vi "Slack OAuth Test.vi"() -> ()   [LabVIEW 2020]
uses:
  Oauth2.Slack/Oauth2.Slack.lvclass
  C:/Data/1_Projects/CIGH_Oauth2/source/Oauth2/Oauth2.lvclass
  Oauth2/Oauth2.lvclass
  <vilib>/LabVIEW Open Source Project/OpenURI/uri/URI.lvclass
  <vilib>/httpClient/LabVIEWHTTPClient.lvlib
panel:
  out "Slack User List":string
  out "HTTP Response Headers":string
  in  "Client Secret":string
  in  "Client ID":string
  out "Slack Access Token":string
  out "error out":errorcluster
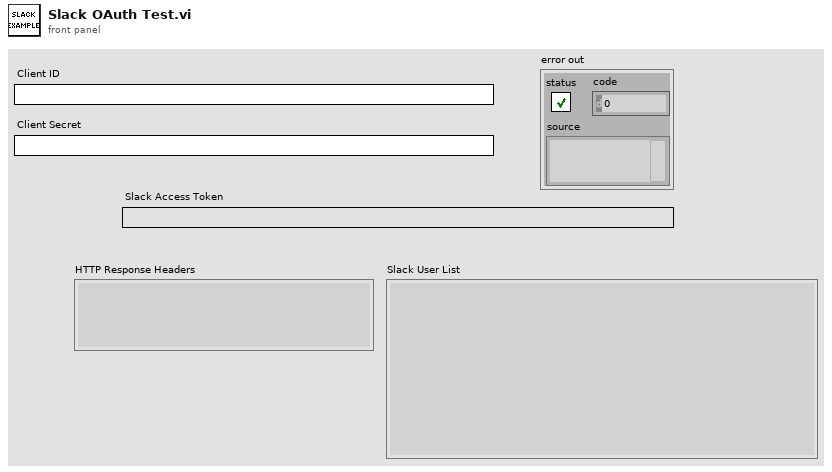
[diagram p1: front panel]
types:
  T1 = typedef "LabVIEWHTTPClient.lvlib/ClientHandle.ctl" = refnum<k1>
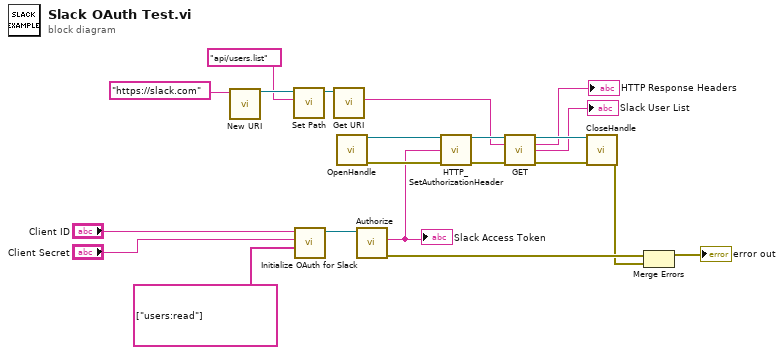
[diagram p0: block diagram]
diagram:
  n1 = call <vilib>:"New URI.vi"("URI"="https://slack.com" ("path")) -> ("URI"=w17:refnum<class "URI.lvclass">)  [unwired: 9 in, 1 out]
  n2 = call <vilib>:"Set Path.vi"("path"="api/users.list", "URI in"=w17) -> ("URI out"=w15:refnum<class "URI.lvclass">)  [unwired: 8 in, 1 out]
  n3 = call "Initialize OAuth for Slack.vi"("Scopes"=string[] ["users:read"], "Client Secret"="Client Secret", "Client ID"="Client ID") -> ("Oauth2.Slack"=w19:refnum<class "Oauth2.Slack.lvclass">)  [unwired: 8 in]
  n4 = call <vilib>:"Get URI.vi"("URI in"=w15) -> ("URI String"=w8:string)  [unwired: 8 in, 2 out]
  n5 = call <vilib>:"OpenHandle.vi"() -> ("client handle out"=w14:T1, "error out"=w13:errorcluster)  [unwired: 14 in]
  n6 = call "Authorize.vi"("Oauth2 in"=w19) -> ("error out"=w3:errorcluster, "Access Token"=w5:string)  [unwired: 8 in, 1 out]
  "Slack Access Token" <- w5
  n7 = call "HTTP_SetAuthorizationHeader.vi"("Client Handle"=w14, "Access Token"=w5, "error in (no error)"=w13) -> ("client handle dup"=w12:T1, "error out"=w11:errorcluster)  [unwired: 11 in]
  n8 = call <vilib>:"GET.vi"("client handle"=w12, "url"=w8, "error in (no error)"=w11) -> ("client handle out"=w10:T1, "headers"=→"HTTP Response Headers":string, "body"=→"Slack User List":string, "error out"=w9:errorcluster)  [unwired: 9 in]
  n9 = call <vilib>:"CloseHandle.vi"("client handle"=w10, "error in (no error)"=w9) -> ("error out"=w1:errorcluster)  [unwired: 13 in]
  n10 = Merge Errors(w3, w1) -> (→"error out":errorcluster)
